vi "题目8.vi"() -> ()   [LabVIEW 2017]
uses:
  <vilib>/Utility/file.llb/Write Delimited Spreadsheet (DBL).vi
  <vilib>/measure/NI_MABase.lvlib
panel:
  out "数组":dbl[](array[numeric])
  out "波形图":waveform(dbl)(graph)
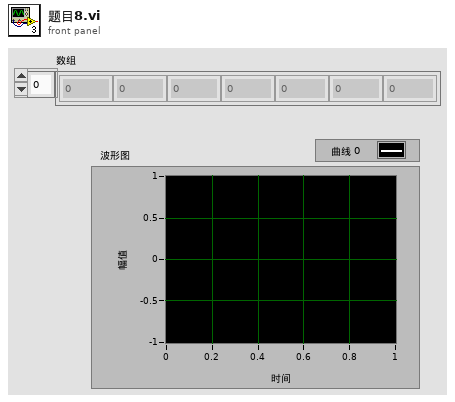
[diagram p1: front panel]
types:
  T1 = enum16{"open", "replace", "create", "open or create", "replace or create", "replace or create with confirmation"}
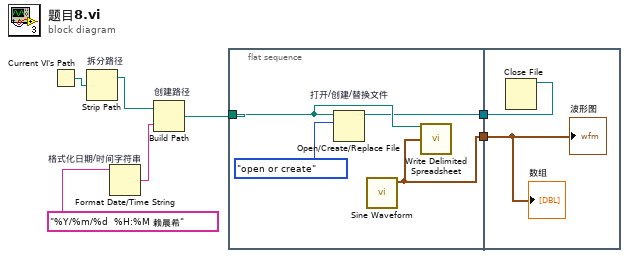
[diagram p0: block diagram]
diagram:
  n1 = Current VI's Path() -> (path=w7:path)
  n2 = Strip Path "拆分路径"(path=w7) -> (stripped path=w6:path)  [unwired: 1 out]
  n3 = Format Date/Time String "格式化日期/时间字符串"(time format string (%c)="%Y/%m/%d  %H:%M 赖晨希" ("时间格式字符串(%c)")) -> (date/time string=w5:string)  [unwired: 2 in]
  n4 = Build Path "创建路径"(base path=w6, name or relative path=w5) -> (appended path=w3:path)
  n5 = flat-sequence {
    tunnel: w3 -> [w11]
    tunnel: [w10] -> w2
    tunnel: [w9] -> w1
    tunnel: w2 -> [w13]
    tunnel: w1 -> [w12]
    frame #0 {
      n6 = Open/Create/Replace File "打开/创建/替换文件"(file path (use dialog)=w11, operation (0:open)=T1."open or create" ("操作(0:open)")) -> (refnum out=w10:refnum<file>)  [unwired: 4 in, 2 out]
      n7 = call <vilib>:"Sine Waveform.vi"() -> ("signal out"=w9:waveform(dbl))  [unwired: 10 in, 1 out]
      n8 = call-poly <vilib>:"Write Delimited Spreadsheet.vi"("file path (dialog if empty)"=w11, "1D data"=w9) -> ()  [unwired: 12 in, 2 out]
    }
    frame #1 {
      n9 = Close File(refnum=w13) -> ()  [unwired: 1 in, 2 out]
      "波形图" <- w12
      "数组" <- w12
    }
  }
